vi "F(e).vi"(7 "Neuron Type":enum16{"Linear", "Sigmoid", "Tangent hyp."}(ring), 10 "Weights":dbl[](array[numeric]), 11 "Inputs":dbl[](array[numeric])) -> (3 "f(e)":dbl)   [LabVIEW 2012]
panel:
  # "Chuck Streb Dec2007"
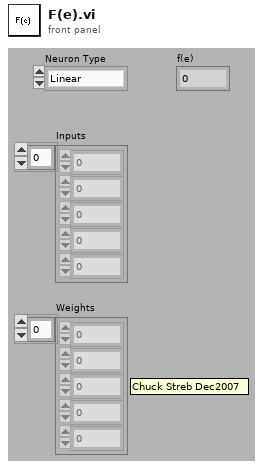
[diagram p1: front panel]
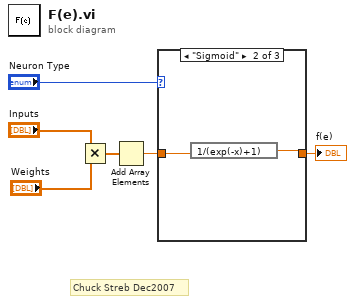
[diagram p0: block diagram]
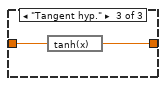
[diagram p3: hidden frame]
diagram:
  # "Chuck Streb Dec2007"
  n1 = Multiply(x="Inputs", y="Weights") -> (x*y=w4:dbl[])
  n2 = Add Array Elements(numeric array=w4) -> (sum=w1:dbl)
  n3 = case shown="\"Sigmoid\"" "Neuron Type" {
    tunnel: w1 -> [w7 w9 w11]
    tunnel: [w7 w8 w10] -> w2
    frame "Linear", Default {
    }
    frame "Sigmoid" {
      n4 = expression code="1/(exp(-x)+1)"(w9) -> (w8:dbl)
    }
    frame "Tangent hyp." {
      n5 = expression code="tanh(x)"(w11) -> (w10:dbl)
    }
  }
  "f(e)" <- w2
